vi "All Variant to numbers.vi"(3 "Error in":errorcluster caption="错误输入", 5 "Variant input":variant[](array[variant])) -> (0 "Error out":errorcluster caption="错误输出", 1 "Var Out":i32[](array[numeric]))   [LabVIEW 2014]
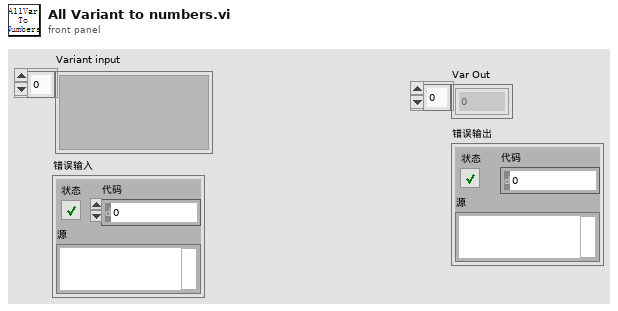
[diagram p1: front panel]
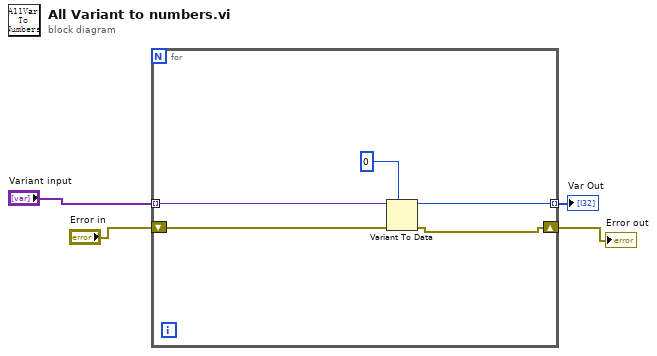
[diagram p0: block diagram]
diagram:
  n1 = for {
    tunnel: "Variant input" -> [w9] mode=indexing
    shift-right: [w7] -> w2
    shift-left: "Error in" -> [w8]
    tunnel: [w5] -> w1 mode=indexing
    n2 = Variant To Data(error in=w8, type=0, Variant=w9) -> (data=w5:i32, error out=w7:errorcluster)
  }
  "Error out" <- w2
  "Var Out" <- w1
